vi "Sort Connections by Pin and Site.vi"(10 "pin sort order":string[](array[string]), 11 "connections":T1[](array[typedef])) -> (3 "sorted connections":T1[](array[typedef]))   [LabVIEW 2020]
uses:
  Connection with Session.ctl
  Connection.ctl
  Connection Sorter By Site/Connection Sorter By Site.lvclass
  185d3de3-35dd-42dd-8dfb-462d9ad0c4ce.vi
  185d3de3-35dd-42dd-8dfb-462d9ad0c4ce.vi/4611cae3-c7be-41e2-9a5e-ea0ae78a7ced.vi
  185d3de3-35dd-42dd-8dfb-462d9ad0c4ce.vi/4611cae3-c7be-41e2-9a5e-ea0ae78a7ced.vi/711a7bad-6791-4773-b8dd-6fbaf24e5b7c.vi
  185d3de3-35dd-42dd-8dfb-462d9ad0c4ce.vi/4611cae3-c7be-41e2-9a5e-ea0ae78a7ced.vi/ab28192a-3d92-42da-8523-74871bf534c0.vi
  185d3de3-35dd-42dd-8dfb-462d9ad0c4ce.vi/4611cae3-c7be-41e2-9a5e-ea0ae78a7ced.vi/d47d084a-d94a-47c5-b962-ca4ced011778.vi
  185d3de3-35dd-42dd-8dfb-462d9ad0c4ce.vi/4611cae3-c7be-41e2-9a5e-ea0ae78a7ced.vi/0d0dd576-019e-4093-8822-9b4bde5edcbe.vi
  185d3de3-35dd-42dd-8dfb-462d9ad0c4ce.vi/4611cae3-c7be-41e2-9a5e-ea0ae78a7ced.vi/148138b5-abcc-4d18-a1cb-fad94e4c517a.vi
  185d3de3-35dd-42dd-8dfb-462d9ad0c4ce.vi/4611cae3-c7be-41e2-9a5e-ea0ae78a7ced.vi/46408cae-4ea5-4f15-ab36-8bc0fd18527a.vi
  185d3de3-35dd-42dd-8dfb-462d9ad0c4ce.vi/4611cae3-c7be-41e2-9a5e-ea0ae78a7ced.vi/b1fbf645-60c9-4d68-8ae9-d3187fe658c2.vi
  185d3de3-35dd-42dd-8dfb-462d9ad0c4ce.vi/4611cae3-c7be-41e2-9a5e-ea0ae78a7ced.vi/5179999f-faab-4e10-925a-f43c3f28d8d8.vi
  185d3de3-35dd-42dd-8dfb-462d9ad0c4ce.vi/4611cae3-c7be-41e2-9a5e-ea0ae78a7ced.vi/14adcb6d-7f20-40e2-b0f4-539fd4458acc.vi
  Connection Sorter By Site/Less Than.vi
  Session Reservation.lvclass
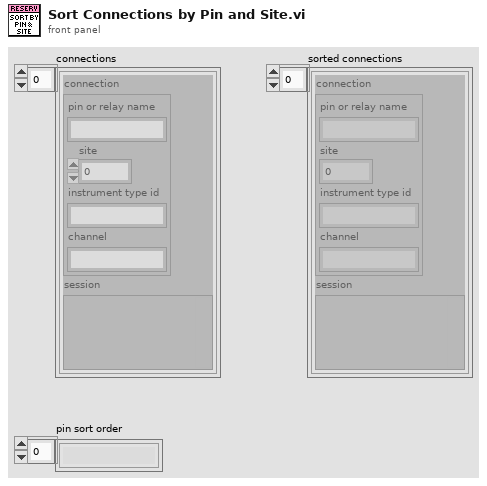
[diagram p1: front panel]
types:
  T1 = typedef "MeasurementLink Session Management.lvlib/Session Reservation.lvclass/Connection with Session.ctl" = cluster{"connection":T2, "session":variant}
  T2 = typedef "MeasurementLink Session Management.lvlib/Session Reservation.lvclass/Connection.ctl" = cluster{"pin or relay name":string, "site":i32, "instrument type id":string, "channel":string}
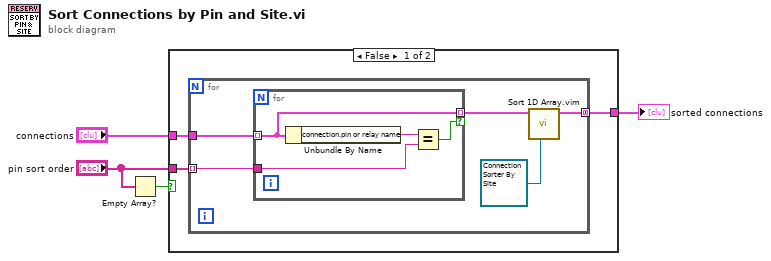
[diagram p0: block diagram]
diagram:
  n1 = Empty Array?(array="pin sort order") -> (empty?=w1:bool)
  n2 = case shown="False" w1 {
    tunnel: "connections" -> [w7 w17]
    tunnel: [w6 w17] -> w3
    tunnel: "pin sort order" -> [w5 _]
    frame False {
      n3 = for {
        tunnel: w7 -> [w12]
        tunnel: w5 -> [w11] mode=indexing
        tunnel: [w8] -> w6 mode=concatenating
        n4 = for {
          tunnel: w12 -> [w14] mode=indexing
          tunnel: w11 -> [w15]
          tunnel: [w14] -> w9 mode=indexing if=w13
          n5 = Unbundle By Name(w14) -> ("connection.pin or relay name"=w16:string)
          n6 = Equal?(x=w16, y=w15) -> (x = y?=w13:bool)
        }
        n7 = call "Sort 1D Array.vim"("less function (built-in <)"=refnum<class "Connection Sorter By Site.lvclass"> refnum ("MeasurementLink Session Management.lvlib:Connection Sorter By Site.lvclass"), "unsorted array"=w9) -> ("sorted array"=w8:T1[])  [unwired: 9 in]
      }
    }
    frame True {
    }
  }
  "sorted connections" <- w3
